vi "SVL AC & DC Level.vi"   [LabVIEW 2017]
doc: "Computes the AC level and DC level of a signal. Wire data to the <B>scaled signal [EU]</B> input to determine the polymorphic instance to use or manually select the instance."
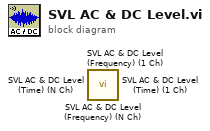
[diagram p0: block diagram]
diagram:
  n1 = call <vilib>:"SVL AC & DC Level (Frequency) (N Ch).vi"() -> ()  [unwired: 14 in, 6 out]
  n2 = call <vilib>:"SVL AC & DC Level (Frequency) (1 Ch).vi"() -> ()  [unwired: 14 in, 6 out]
  n3 = call <vilib>:"SVL AC & DC Level (Time) (N Ch).vi"() -> ()  [unwired: 14 in, 6 out]
  n4 = call <vilib>:"SVL AC & DC Level (Time) (1 Ch).vi"() -> ()  [unwired: 14 in, 6 out]
